vi "S_R.vi"() -> ()   [LabVIEW 2018]
panel:
  out "Numeric":dbl
  out "Numeric 2":i32
  out "Numeric 3":i32
  out "Numeric 4":i32
  out "Numeric 5":i32
  in  "stop":bool
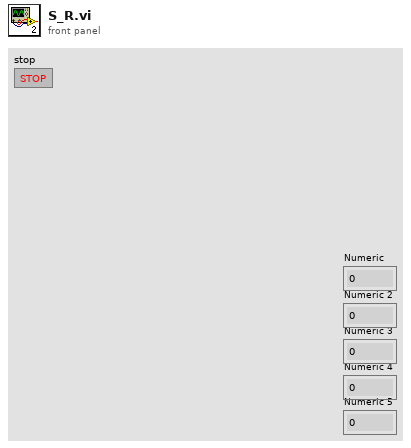
[diagram p1: front panel]
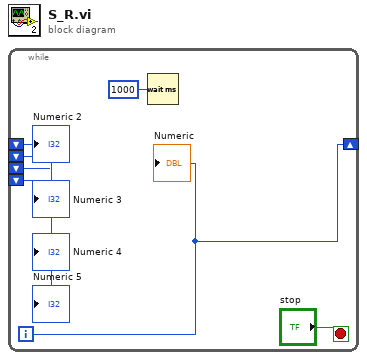
[diagram p0: block diagram]
diagram:
  n1 = while {
    shift-right: [w6] -> _
    shift-left: _ -> [w5]
    shift-left: _ -> [w4]
    shift-left: _ -> [w3]
    shift-left: _ -> [w2]
    i -> [w6]
    stop <- "stop" stop-if-true
    n2 = Wait (ms)(milliseconds to wait=u32 1000) -> ()  [unwired: 1 out]
    "Numeric" <- w6
    "Numeric 2" <- w5
    "Numeric 3" <- w4
    "Numeric 4" <- w3
    "Numeric 5" <- w2
  }
